vi "Inverse Real FFT(half complex).vi"(0 "FFT {X}":dbl[](array[numeric]) format="%0.2f") -> (1 "X":dbl[](array[numeric]) format="%0.2f", 2 "error":i32)   [LabVIEW 2014, in "NI_AALPro.lvlib"]
doc: "Computes the Real Fast Fourier Transform (FFT) or the Real Discrete Fourier Transform (DFT) of the input sequence <B>X</B>."
uses:
  NI_AALPro.lvlib
  lvanlys.dll
panel:
  # "Inverse Real FFT (Half Complex)"
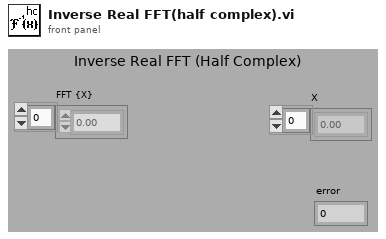
[diagram p1: front panel]
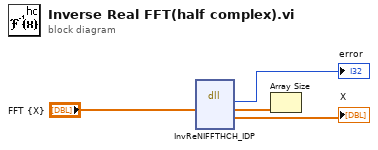
[diagram p0: block diagram]
diagram:
  n1 = dll-call lib="C:/Program Files (x86)/National Instruments/LabVIEW 2014/resource/lvanlys.*" fn="InvReNIFFTHCH_IDP"("xH"="FFT {X}") -> ("return type"=→"error":i32, "xH"=w1:dbl[], "yH"=→"X":dbl[])  [unwired: 6 in, 2 out]
  n2 = Array Size(array=w1) -> ()  [unwired: 1 out]
